vi "Weather Stations Data (JSON) To LVData.vi"(8 "error in (no error)":errorcluster, 11 "Weather Stations Data (JSON)":string) -> (0 "error out":errorcluster, 3 "Data":T9)   [LabVIEW 2020, in "Netatmo-WeatherStation.lvlib"]
uses:
  Netatmo-WeatherStation.lvlib
  TypeDefs/body.ctl
  TypeDefs/devices.items.ctl
  TypeDefs/place.ctl
  TypeDefs/devices.dashboard_data.ctl
  TypeDefs/modules.items.ctl
  TypeDefs/modules.dashboard_data.ctl
  TypeDefs/user.ctl
  TypeDefs/administrative.ctl
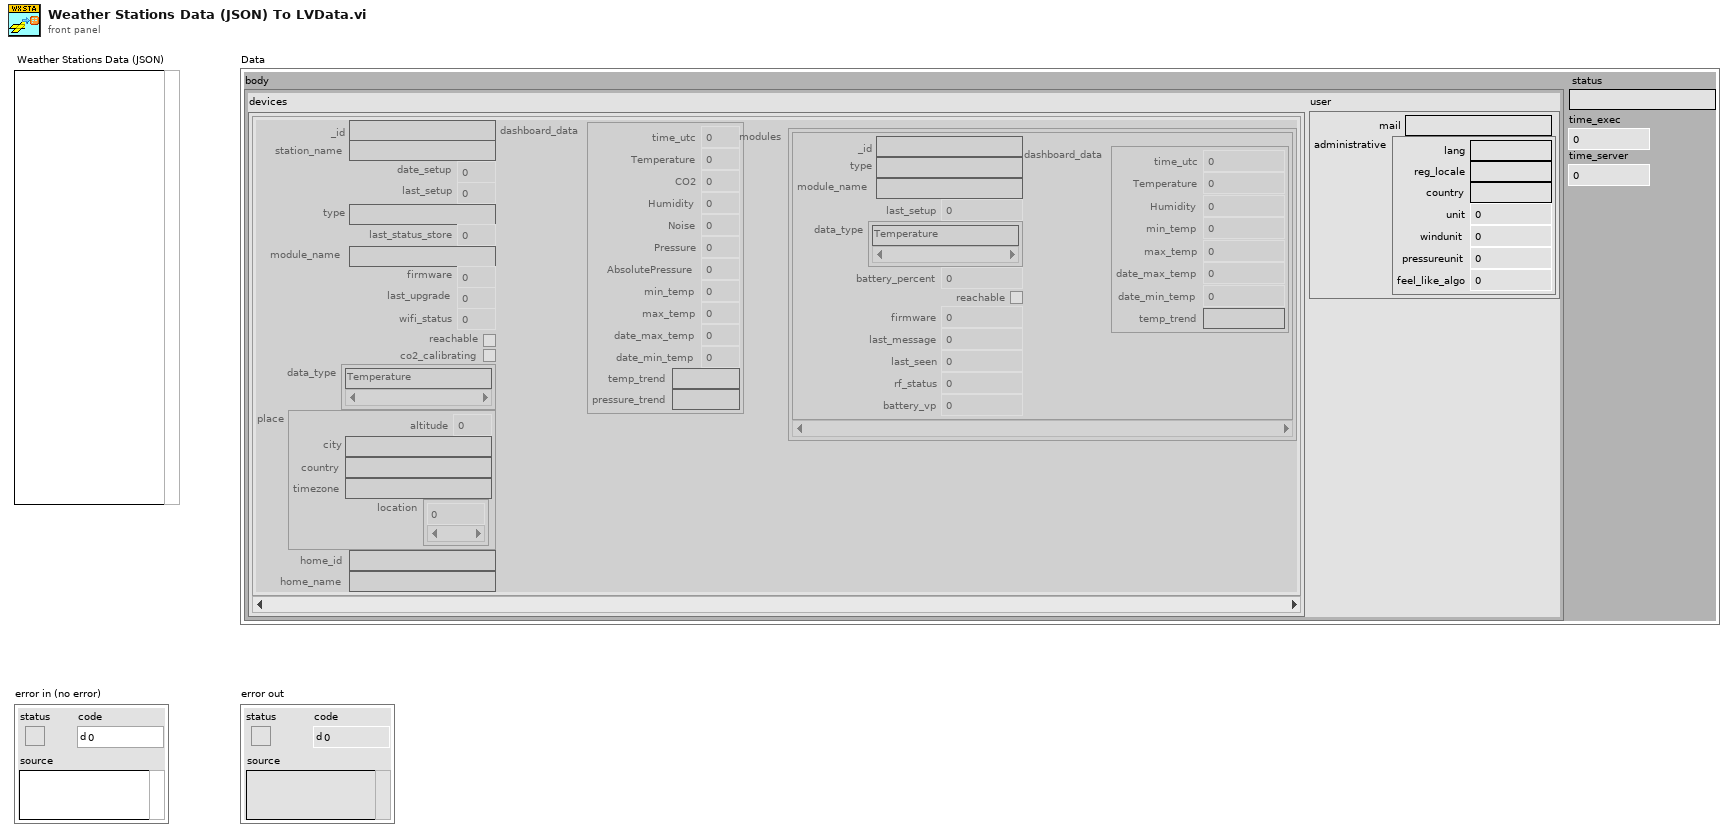
[diagram p1: front panel]
types:
  T1 = typedef "Netatmo-WeatherStation.lvlib/body.ctl" = cluster{"devices":T2[], "user":T7}
  T2 = typedef "Netatmo-WeatherStation.lvlib/devices.items.ctl" = cluster{"_id":string, "station_name":string, "date_setup":dbl, "last_setup":dbl, "type":string, "last_status_store":dbl, "module_name":string, "firmware":dbl, "last_upgrade":dbl, "wifi_status":dbl, "reachable":bool, "co2_calibrating":bool, "data_type":string[], "place":T3, "home_id":string, "home_name":string, "dashboard_data":T4, "modules":T5[]}
  T3 = typedef "Netatmo-WeatherStation.lvlib/place.ctl" = cluster{"altitude":dbl, "city":string, "country":string, "timezone":string, "location":dbl[]}
  T4 = typedef "Netatmo-WeatherStation.lvlib/devices.dashboard_data.ctl" = cluster{"time_utc":dbl, "Temperature":dbl, "CO2":dbl, "Humidity":dbl, "Noise":dbl, "Pressure":dbl, "AbsolutePressure":dbl, "min_temp":dbl, "max_temp":dbl, "date_max_temp":dbl, "date_min_temp":dbl, "temp_trend":string, "pressure_trend":string}
  T5 = typedef "Netatmo-WeatherStation.lvlib/modules.items.ctl" = cluster{"_id":string, "type":string, "module_name":string, "last_setup":dbl, "data_type":string[], "battery_percent":dbl, "reachable":bool, "firmware":dbl, "last_message":dbl, "last_seen":dbl, "rf_status":dbl, "battery_vp":dbl, "dashboard_data":T6}
  T6 = typedef "Netatmo-WeatherStation.lvlib/modules.dashboard_data.ctl" = cluster{"time_utc":dbl, "Temperature":dbl, "Humidity":dbl, "min_temp":dbl, "max_temp":dbl, "date_max_temp":dbl, "date_min_temp":dbl, "temp_trend":string}
  T7 = typedef "Netatmo-WeatherStation.lvlib/user.ctl" = cluster{"mail":string, "administrative":T8}
  T8 = typedef "Netatmo-WeatherStation.lvlib/administrative.ctl" = cluster{"lang":string, "reg_locale":string, "country":string, "unit":dbl, "windunit":dbl, "pressureunit":dbl, "feel_like_algo":dbl}
  T9 = cluster{"body":T1, "status":string, "time_exec":dbl, "time_server":dbl}
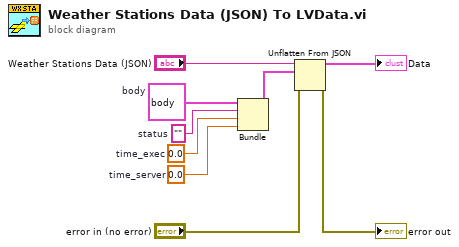
[diagram p0: block diagram]
diagram:
  w4 = 0.0  # time_server
  w5 = 0.0  # time_exec
  w6 = ""  # status
  w7 = T1 {"devices"=[], "user"={"mail"="", "administrative"={"lang"="", "reg_locale"="", "country"="", "unit"=0.0, "windunit"=0.0, "pressureunit"=0.0, "feel_like_algo"=0.0}}}  # body
  n1 = Bundle("body"=w7, "status"=w6, "time_exec"=w5, "time_server"=w4) -> (w2:T9)  [unwired: 1 in]
  n2 = Unflatten From JSON(JSON string="Weather Stations Data (JSON)", type and defaults=w2, error in (no error)="error in (no error)") -> (value=→"Data":T9, error out=→"error out":errorcluster)  [unwired: 4 in]
